vi "Clear I2C Monitor Table.vi"(5 "# TXNS IN TABLE Ref":refnum<vi>, 7 "I2C Table Ref":refnum<vi>, 8 "error in (no error)":errorcluster) -> (0 "error out":errorcluster)   [LabVIEW 2025, in "I2C Bus Monitor UI.lvlib"]
uses:
  I2C Bus Monitor UI.lvlib
  <vilib>/Utility/miscctls.llb/LVRowAndColumnTypeDef.ctl
  Table Buffer - Flush.vi
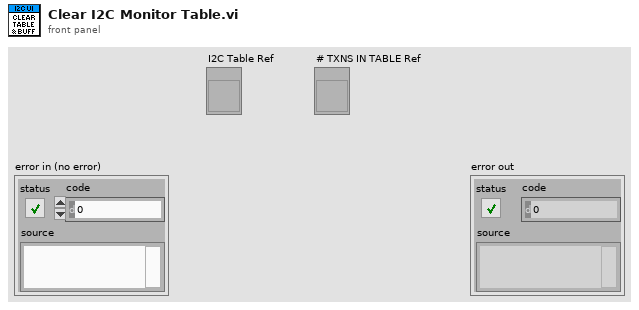
[diagram p1: front panel]
types:
  T1 = typedef "LVRowAndColumnTypeDef.ctl" = cluster{"Row":i32, "Column":i32}
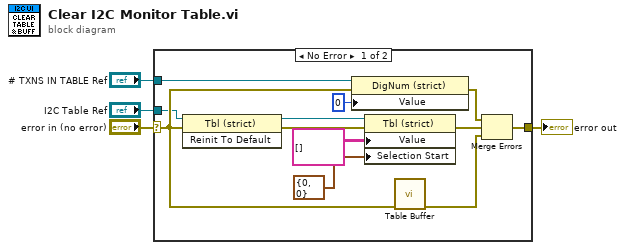
[diagram p0: block diagram]
diagram:
  n1 = case shown="No Error" "error in (no error)" {
    selector: "error in (no error)" -> [w8 w17]
    tunnel: "I2C Table Ref" -> [w7 _]
    tunnel: [w10 w17] -> w2
    tunnel: "# TXNS IN TABLE Ref" -> [w15 _]
    frame No Error {
      n2 = invoke class="Tbl (strict)" method="Reinit To Default"(reference=w7, error in=w8) -> (reference out=w5:refnum<vi>, error out=w6:errorcluster)  [unwired: 1 in, 1 out]
      n3 = property on="Property Node" class="DigNum (strict)"(reference=w15, error in=w8, "Value"=0) -> (error out=w12:errorcluster)  [unwired: 1 out]
      n4 = property on="Property Node" class="Tbl (strict)"(reference=w5, error in=w6, "Value"=string[][] [], "Selection Start"=T1 {"Row"=0, "Column"=0}) -> (error out=w13:errorcluster)  [unwired: 1 out]
      n5 = call-poly "Table Buffer.vi"("error in (no error)"=w8) -> ("error out"=w11:errorcluster)  [unwired: 10 in]
      n6 = Merge Errors(w12, w13, w11) -> (w10:errorcluster)
    }
    frame Error {
    }
  }
  "error out" <- w2
